vi "TablaTD.vi"(8 "error in (no error)":errorcluster, 9 "fila":i32, 10 "NivelMedido":dbl, 11 "Prueba21_1 in":refnum<class "Prueba21.lvclass">) -> (0 "error out":errorcluster, 3 "Prueba21_1 out":refnum<class "Prueba21.lvclass">)   [LabVIEW 2019, in "Prueba21.lvclass"]
uses:
  Prueba21.lvclass
  Prueba21.lvclass/Prueba21.ctl
  Prueba/Prueba.lvclass
panel:
  out "array_dB":string[](array[string])
  out "array_dB (num)":dbl[](array[numeric])
  out "prom_dB":dbl
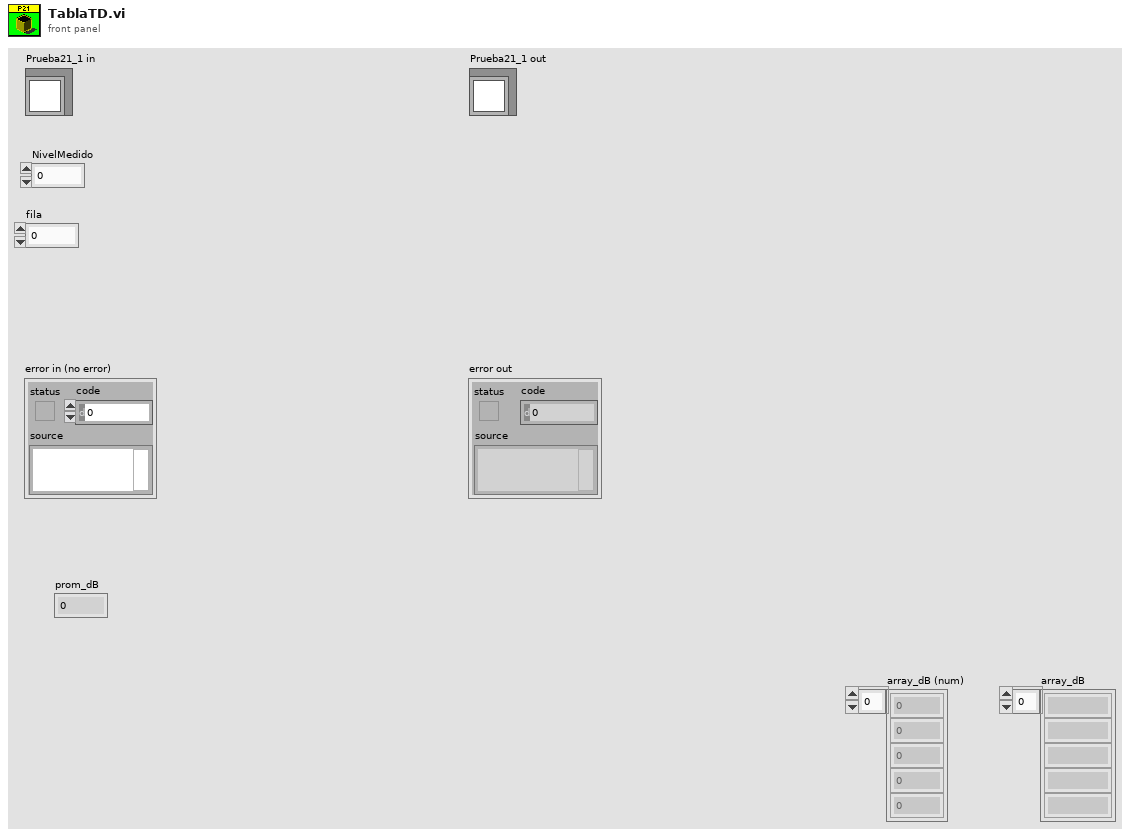
[diagram p1: front panel]
types:
  T1 = cluster{"ControlName":string, "ControlReference":refnum<vi>}[]
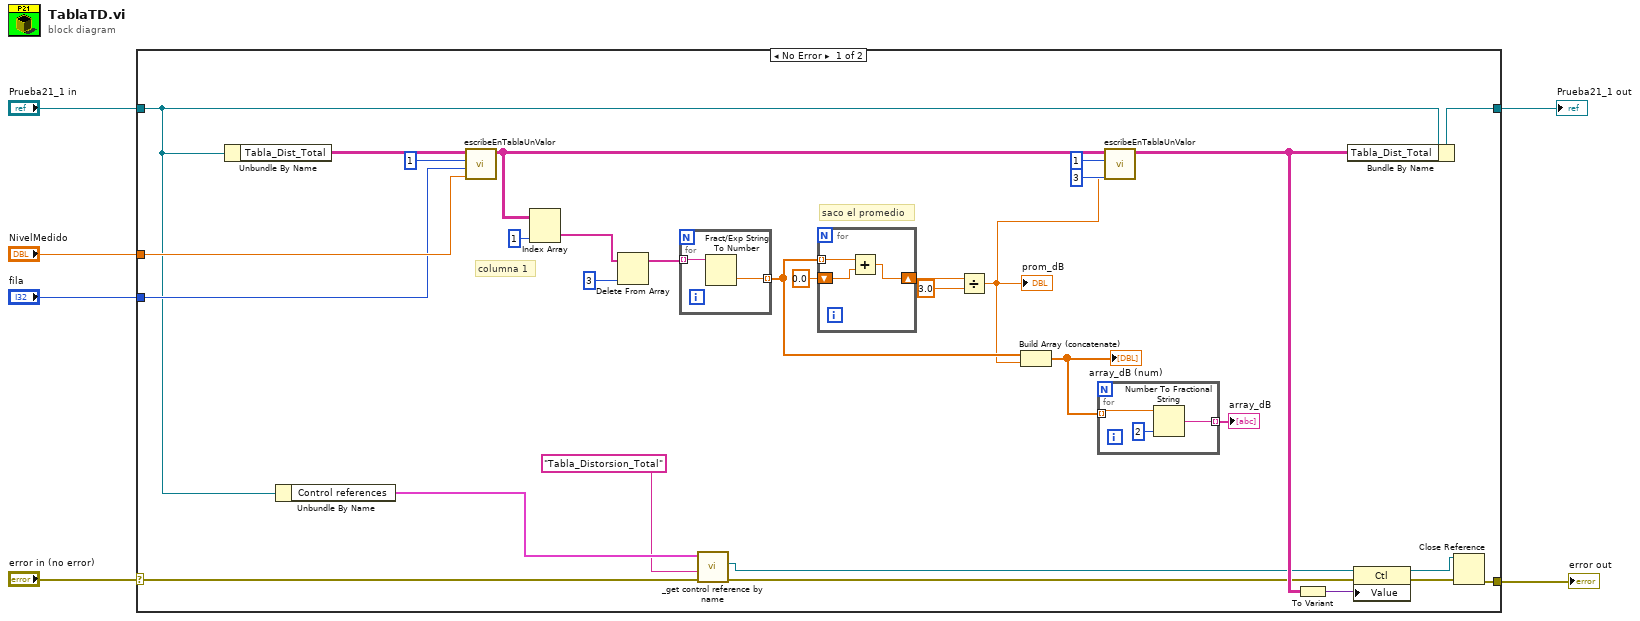
[diagram p0: block diagram]
diagram:
  n1 = case shown="No Error" "error in (no error)" {
    selector: "error in (no error)" -> [w15 w46]
    tunnel: [w10 w46] -> w5
    tunnel: [w21 w45] -> w3
    tunnel: "Prueba21_1 in" -> [w14 w45]
    tunnel: "NivelMedido" -> [w20 _]
    tunnel: "fila" -> [w19 _]
    frame No Error {
      # "columna 1"
      # "saco el promedio"
      n2 = Unbundle By Name(w14) -> ("Tabla_Dist_Total"=w36:string[][])
      n3 = Unbundle By Name(w14) -> ("Control references"=w17:T1)
      n4 = call "escribeEnTablaUnValor.vi"("element"=w20, "fila"=w19, "col"=1, "tabla in"=w36) -> ("tabla out"=w27:string[][])  [unwired: 7 in]
      n5 = Index Array "Index Array"(array=w27, index (col)=1 ("disabled index (col)")) -> (element=w30:string[])  [unwired: 1 in]
      n6 = Delete From Array(array=w30, index=3) -> (array with subset deleted=w28:string[])  [unwired: 1 in, 1 out]
      n7 = for {
        tunnel: w28 -> [w44] mode=indexing
        tunnel: [w43] -> w24 mode=indexing
        n8 = Fract/Exp String To Number(string=w44) -> (number=w43:dbl)  [unwired: 3 in, 1 out]
      }
      n9 = call "_get control reference by name.vi"("error in (no error)"=w15, "Control name"="Tabla_Distorsion_Total", "Control references"=w17) -> ("error out"=w8:errorcluster, "Ctl Refnum"=w7:refnum<vi>)  [unwired: 3 in]
      n10 = for {
        shift-right: [w40] -> w32
        shift-left: 0.0 ("number") -> [w41]
        tunnel: w24 -> [w42] mode=indexing
        n11 = Add(x=w42, y=w41) -> (x+y=w40:dbl)
      }
      n12 = Divide(x=w32, y=3.0) -> (x/y=w18:dbl)
      "prom_dB" <- w18
      n13 = Build Array (concatenate)(w24, w18) -> (w23:dbl[])
      "array_dB (num)" <- w23
      n14 = for {
        tunnel: w23 -> [w39] mode=indexing
        tunnel: [w37] -> w22 mode=indexing
        n15 = Number To Fractional String(number=w39, precision (6)=i16 2) -> (F-format string=w37:string)  [unwired: 2 in]
      }
      "array_dB" <- w22
      n16 = call "escribeEnTablaUnValor.vi"("element"=w18, "fila"=3, "col"=1, "tabla in"=w27) -> ("tabla out"=w9:string[][])  [unwired: 7 in]
      n17 = To Variant(anything=w9) -> (Variant=w13:variant)
      n18 = Bundle By Name(cluster=w14, "Tabla_Dist_Total"=w9) -> (w21:refnum<class "Prueba21.lvclass">)
      n19 = property on="Property Node" class="Ctl"(reference=w7, error in=w8, "Value"=w13) -> (reference out=w12:refnum<vi>, error out=w11:errorcluster)
      n20 = Close Reference(reference=w12, error in (no error)=w11) -> (error out=w10:errorcluster)
    }
    frame Error {
    }
  }
  "error out" <- w5
  "Prueba21_1 out" <- w3
